vi "Main.vi"() -> ()   [LabVIEW 2020]
doc: "This template is for the Queued Message Handler design pattern.\n\nThe Event Handling Loop generates messages based on user interface actions.\n\nThe Message Handling Loop processes messages generated by the Event Handling Loop, or by other messages. The messages are string values, so new messages can be added easily to the Message Cases case structure in the Message Handling Loop. Each message cluster can also provide an optional value for Message Data, which is a variant that can be converted to whatever message-specific data is required."
uses:
  controls/UI Data.ctl
  support/Message Queue/Message Cluster.ctl
  <vilib>/DAQmx/read.llb/DAQmx Read (Analog 1D DBL 1Chan NSamp).vi
  <extravilib>/ChannelInstances/Messenger-t'Message Queue.lvlib-Message Cluster.ctl'/Write With Abort.vi
  <extravilib>/ChannelInstances/Messenger-t'Message Queue.lvlib-Message Cluster.ctl'/Instantiate.vi
  <extravilib>/ChannelInstances/Messenger-t'Message Queue.lvlib-Message Cluster.ctl'/Endpoint.vi
  <extravilib>/ChannelInstances/Event Messenger-bool/Instantiate.vi
  <extravilib>/ChannelInstances/Event Messenger-bool/))Channel.vi
  <vilib>/DAQmx/create/channels.llb/DAQmx Create Channel (AI-Voltage-Basic).vi
  <vilib>/DAQmx/configure/timing.llb/DAQmx Timing (Sample Clock).vi
  <vilib>/DAQmx/miscellaneous.llb/DAQmx Fill In Error Info.vi
  <vilib>/ErrorRing/Error Ring.xnode
  <extravilib>/ChannelInstances/Event Messenger-bool.lvlib
  support/Message Queue/Message Queue.lvlib
  <extravilib>/ChannelInstances/Messenger-t'Message Queue.lvlib-Message Cluster.ctl'.lvlib
  <resource>/objmgr/daqmx.rc
panel:
  out "Actual Sample Rate":dbl
  in  "Threshold":dbl=4.0
  in  "Analyze Signal":bool
  in  "Sample Rate":dbl=1000.0
  in  "Generate Signal":bool
  out "Threshold Exceeded?":bool
  out "RMS Result":dbl
  out "Current Consumer State":string
  out "Waveform Graph":dbl[](graph)
  in  "Exit":bool
  # "These controls have associated \"Value Changed\" events configured in the Event Structure on the diagram.\n\nReplace them (and reconfigure the Event Structure) with the controls you need for your application."
  # "This template is for the Queued Message Handler design pattern.\n\nSee the block diagram for more information on how to use this template."
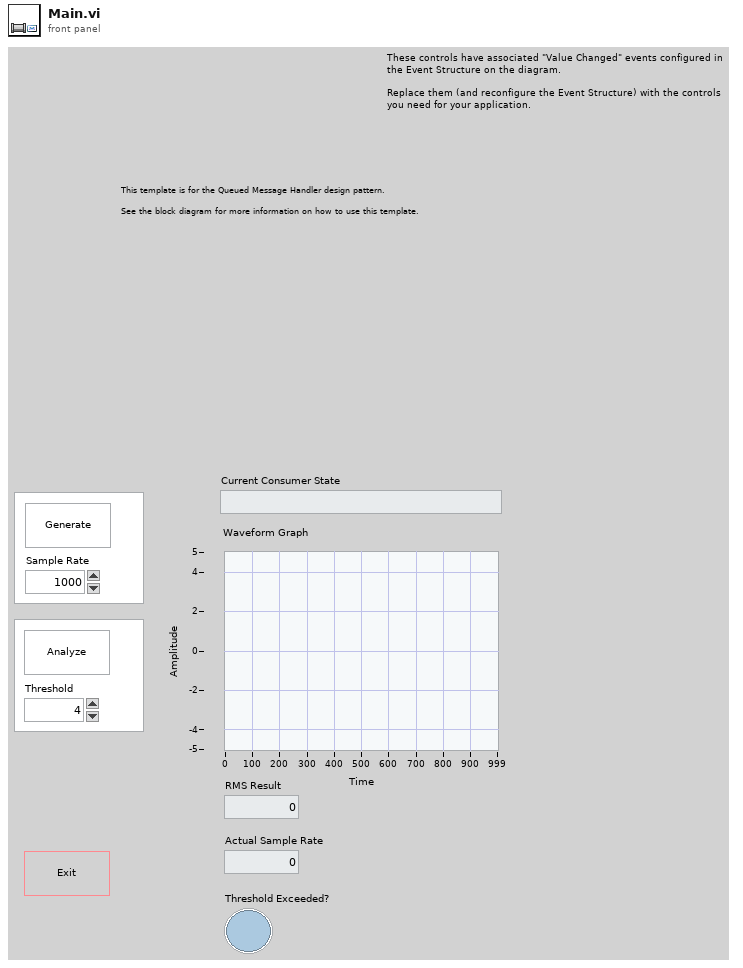
[diagram p1: front panel]
types:
  T1 = typedef "Message Queue.lvlib/Message Cluster.ctl" = cluster{"Message":string, "Message Data":variant}
  T2 = typedef "UI Data.ctl" = cluster{"Message":string, "Message Data":u32}
  T3 = typedef "Messenger-t'Message Queue.lvlib-Message Cluster.ctl'.lvlib/))Channel.ctl" = refnum<queue>
  T4 = typedef "Event Messenger-bool.lvlib/))Channel.ctl" = refnum<queue>
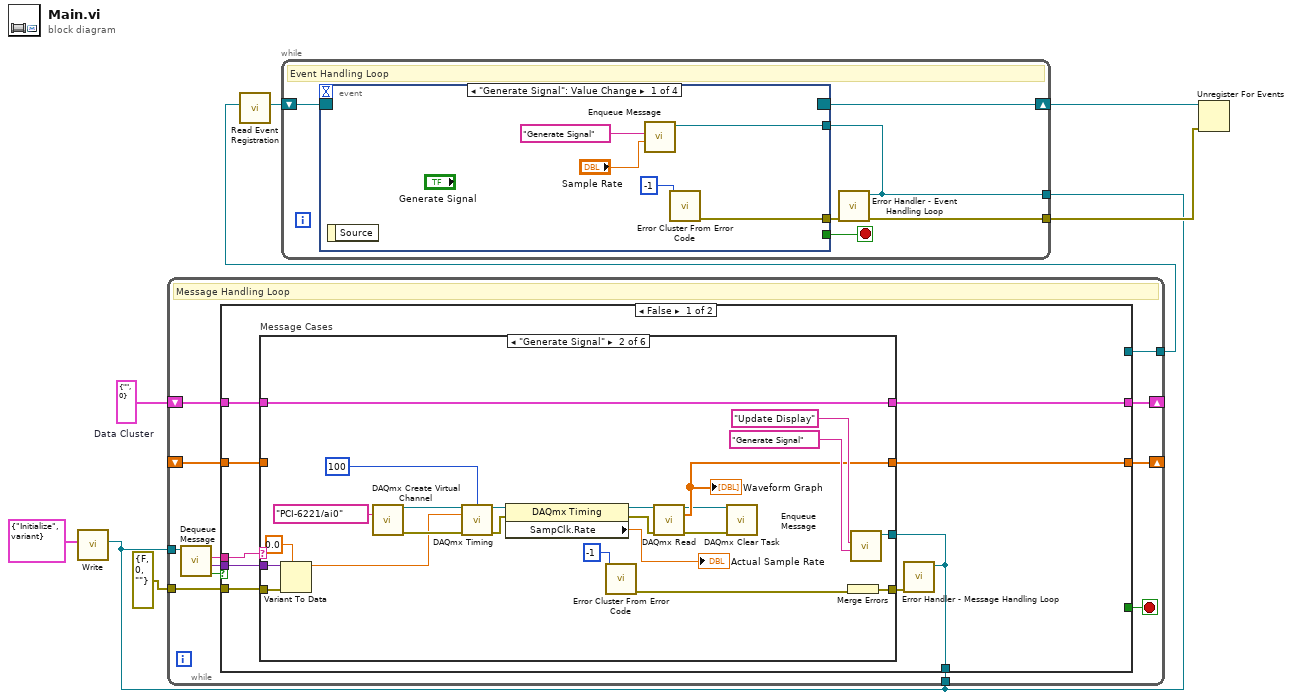
[diagram p0: block diagram]
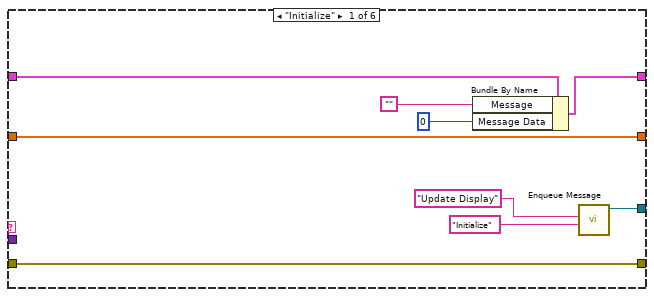
[diagram p2: hidden frame]
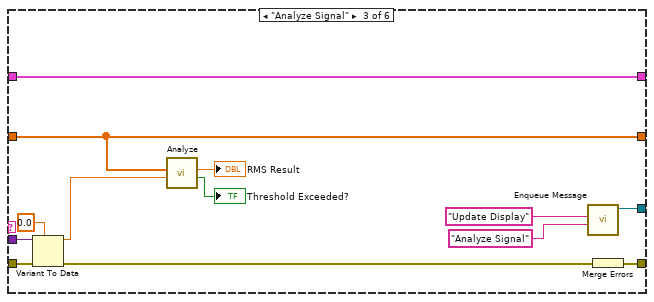
[diagram p3: hidden frame]
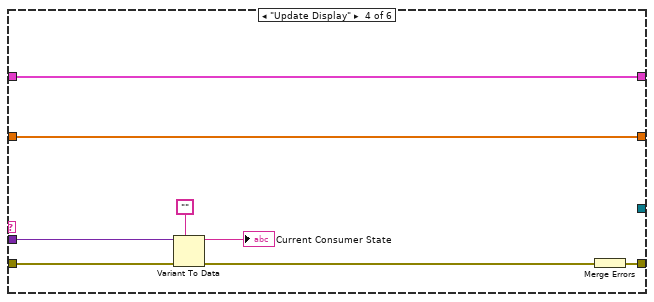
[diagram p4: hidden frame]
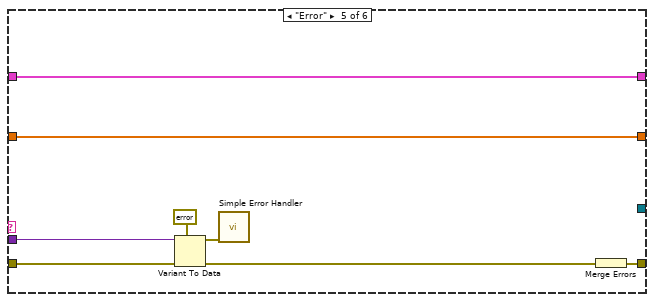
[diagram p5: hidden frame]
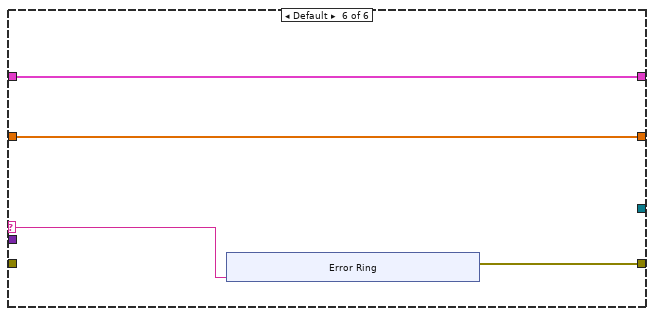
[diagram p6: hidden frame]
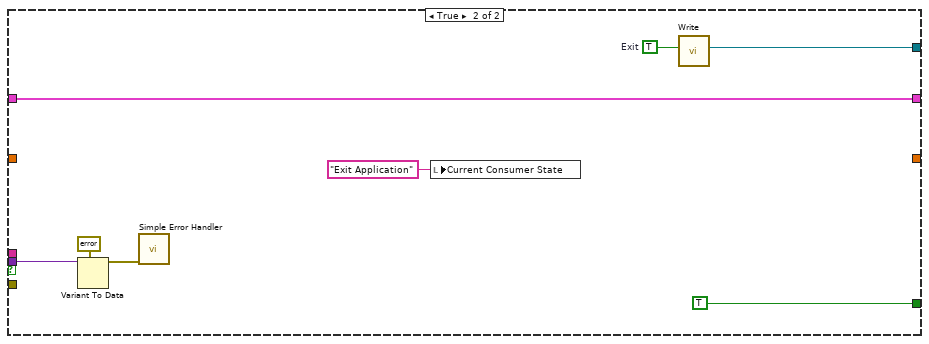
[diagram p7: hidden frame]
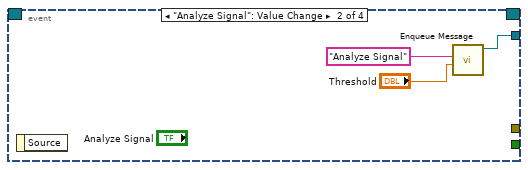
[diagram p8: hidden frame]
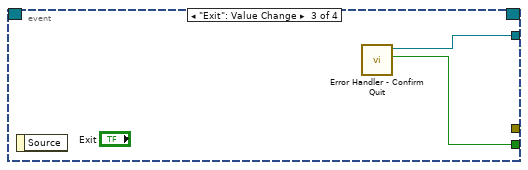
[diagram p9: hidden frame]
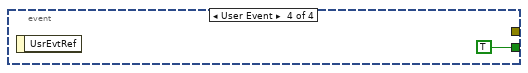
[diagram p10: hidden frame]
diagram:
  w7 = T2 {"Message"="", "Message Data"=0}  # Data Cluster
  n1 = call <extravilib>:"Write.vi"("element"=T1 {"Message"="Initialize", "Message Data"=variant}) -> ("channel"=w2:T3)  [unwired: 8 in, 2 out]
  n2 = while {
    shift-right: [w19] -> _
    shift-left: w7 -> [w20]
    tunnel: [w17] -> w5
    tunnel: w2 -> [w14]
    tunnel: errorcluster {"status"=FALSE, "code"=0, "source"=""} ("error IO") -> [w16]
    tunnel: w2 -> [w15]
    shift-right: [w10] -> _
    shift-left: _ -> [w9]
    stop <- w18 stop-if-true
    # "Message Handling Loop"
    n3 = call "Dequeue Message.vi"("channel"=w14) -> ("channel aborted"=w11:bool, "message data"=w12:variant, "message"=w13:string)  [unwired: 8 in]
    n4 = case shown="False" w11 {
      tunnel: w20 -> [w29 w108]
      tunnel: [w28 w108] -> w19
      tunnel: [_ TRUE] -> w18
      tunnel: [_ w103] -> w17
      tunnel: w13 -> [w26 _]
      tunnel: w12 -> [w25 w105]
      tunnel: w16 -> [w24 _]
      tunnel: [w23 _] -> w15
      tunnel: [w22 _] -> w10
      tunnel: w9 -> [w21 _]
      frame False {
        n5 = case "Message Cases" shown="\"Generate Signal\"" w26 {
          selector: w26 -> [_ _ _ _ _ w92]
          tunnel: w24 -> [w36 w47 w66 w80 w90 _]
          tunnel: [w36 w60 w73 w81 w84 w93] -> w27
          tunnel: w29 -> [w38 w61 w74 w82 w89 w94]
          tunnel: [w37 w61 w74 w82 w89 w94] -> w28
          tunnel: w25 -> [_ w49 w65 w79 w88 _]
          tunnel: [w33 w59 w72 _ _ _] -> w23
          tunnel: [w30 w56 w68 w76 w83 w91] -> w22
          tunnel: w21 -> [w30 _ w68 w76 w83 w91]
          frame "Initialize" {
            # "Initialize - All initialization work should take place in this message, since other loops can potentially enqueue messages that execute immediately after this one."
            n6 = Bundle By Name(cluster=w38, "Message"="", "Message Data"=u32 0 ("Numeric <Replace Me>")) -> (w37:T2)
            n7 = call "Enqueue Message.vi"("data (empty)"="Initialize" ("Initial Message"), "message"="Update Display" ("Message")) -> ("channel"=w33:T3)  [unwired: 9 in]
          }
          frame "Generate Signal" {
            # "Something - Replace this message with functionality for your own application."
            n8 = Variant To Data(error in=w47, type=0.0, Variant=w49) -> (data=w46:dbl)  [unwired: 1 out]
            n9 = call-poly <vilib>:"DAQmx Create Virtual Channel.vi"("physical channels"=tag "PCI-6221/ai0") -> ("task out"=w55:refnum<k21>, "error out"=w54:errorcluster)  [unwired: 13 in]
            n10 = call-poly <vilib>:"DAQmx Timing.vi"("task/channels in"=w55, "samples per channel"=100, "rate"=w46, "error in"=w54) -> ("task out"=w45:refnum<k21>, "error out"=w44:errorcluster)  [unwired: 10 in]
            n11 = property class="DAQmx Timing"(reference=w45, error in=w44) -> (reference out=w43:refnum<k21>, error out=w42:errorcluster, "SampClk.Rate"=→"Actual Sample Rate":dbl)
            n12 = call <vilib>:"Error Cluster From Error Code.vi"("error code (0)"=-1) -> ("error out"=w39:errorcluster)  [unwired: 8 in]
            n13 = call-poly <vilib>:"DAQmx Read.vi"("task/channels in"=w43, "error in"=w42) -> ("task out"=w53:refnum<k21>, "data"=w56:dbl[], "error out"=w52:errorcluster)  [unwired: 11 in]
            "Waveform Graph" <- w56
            n14 = call <vilib>:"DAQmx Clear Task.vi"("task in"=w53, "error in"=w52) -> ()  [unwired: 13 in, 1 out]
            n15 = Merge Errors(w39) -> (w60:errorcluster)
            n16 = call "Enqueue Message.vi"("data (empty)"="Generate Signal" ("\"Do Something\" button pressed"), "message"="Update Display" ("Message")) -> ("channel"=w59:T3)  [unwired: 9 in]
          }
          frame "Analyze Signal" {
            # "Something Else - Replace this message with functionality for your own application."
            n17 = Variant To Data(error in=w66, type=0.0, Variant=w65) -> (data=w63:dbl, error out=w64:errorcluster)
            n18 = call "Analyze.vi"("Threshold (rms)"=w63, "Data (1D DBL)"=w68) -> ("Threshold Exceeded?"=→"Threshold Exceeded?":bool, "RMS Result"=→"RMS Result":dbl)  [unwired: 8 in]
            n19 = call "Enqueue Message.vi"("data (empty)"="Analyze Signal" ("\"Do Something Else\" button pressed"), "message"="Update Display" ("Message")) -> ("channel"=w72:T3)  [unwired: 9 in]
            n20 = Merge Errors(w64) -> (w73:errorcluster)
          }
          frame "Update Display" {
            # "Update Display - Convert the message data to a string to display in the Data Display indicator."
            n21 = Variant To Data(error in=w80, type="", Variant=w79) -> (data=→"Current Consumer State":string, error out=w77:errorcluster)
            n22 = Merge Errors(w77) -> (w81:errorcluster)
          }
          frame "Error" {
            # "Error - Display an error dialog. This message is sent by the \"Error Handler\" VIs at the end of other loops in this application."
            n23 = Variant To Data(error in=w90, type=errorcluster {"status"=FALSE, "code"=0, "source"=""} ("error constant"), Variant=w88) -> (data=w86:errorcluster, error out=w85:errorcluster)
            n24 = call <vilib>:"Simple Error Handler.vi"("error in (no error)"=w86) -> ()  [unwired: 4 in, 5 out]
            n25 = Merge Errors(w85) -> (w84:errorcluster)
          }
          frame Default {
            # "'Default' case only runs if there is a message that isn't defined in any of the other cases.  Output a programming error."
            n26 = xnode "Error Ring"("parameter 0"=w92) -> ("error out"=w93:errorcluster)
          }
        }
        n27 = call "Error Handler - Message Handling Loop.vi"("channel"=w23, "error in (no error)"=w27) -> ()  [unwired: 9 in, 1 out]
      }
      frame True {
        w104 = TRUE  # Exit
        n28 = Variant To Data(type=errorcluster {"status"=FALSE, "code"=0, "source"=""} ("error constant"), Variant=w105) -> (data=w106:errorcluster)  [unwired: 1 in, 1 out]
        n29 = call <vilib>:"Simple Error Handler.vi"("error in (no error)"=w106) -> ()  [unwired: 4 in, 5 out]
        n30 = local write "Current Consumer State"("Exit Application" ("Exit Application")) -> ()
        n31 = call <extravilib>:"Write.vi"("element"=w104) -> ("channel"=w103:T4)  [unwired: 9 in, 1 out]
      }
    }
  }
  n32 = call <extravilib>:"Read Event Registration.vi"("channel"=w5) -> ("event registration refnum"=w4:refnum<event-registration>)  [unwired: 10 in]
  n33 = while {
    shift-right: [w114] -> w8
    shift-left: w4 -> [w115]
    tunnel: [w112] -> w6
    tunnel: w2 -> [w111]
    stop <- w113 stop-if-true
    # "Event Handling Loop"
    n34 = event shown="[0] \"Generate Signal\": Value Change" {
      selector: w115 -> [_ _ _ _]
      dyn-events: [_ _ _ _] -> w114
      timeout: _ -> [_ _ _ _]
      tunnel: [_ _ w124 TRUE ("Discard?")] -> w113
      tunnel: [w120 w123 w125 _] -> w111
      tunnel: [w116 _ _ _] -> w110
      event "Generate Signal": Value Change {
        n35 = event-data() -> ()  [unwired: 1 in, 1 out]
        n36 = call "Enqueue Message.vi"("data (empty)"="Sample Rate", "message"="Generate Signal" ("Message")) -> ("channel"=w120:T3)  [unwired: 9 in]
        n37 = call <vilib>:"Error Cluster From Error Code.vi"("error code (0)"=-1) -> ("error out"=w116:errorcluster)  [unwired: 8 in]
      }
      event "Analyze Signal": Value Change {
        n38 = event-data() -> ()  [unwired: 1 in, 1 out]
        n39 = call "Enqueue Message.vi"("data (empty)"="Threshold", "message"="Analyze Signal" ("Message")) -> ("channel"=w123:T3)  [unwired: 9 in]
      }
      event "Exit": Value Change {
        n40 = event-data() -> ()  [unwired: 1 in, 1 out]
        n41 = call "Error Handler - Confirm Quit.vi"() -> ("exit confirmed"=w124:bool, "channel"=w125:T3)  [unwired: 10 in]
      }
      event User Event {
        n42 = event-data() -> ()  [unwired: 1 in, 1 out]
      }
    }
    n43 = call "Error Handler - Event Handling Loop.vi"("channel"=w111, "error in (no error)"=w110) -> ("dup error in"=w112:errorcluster)  [unwired: 9 in]
  }
  n44 = Unregister For Events(event registration refnum=w8, error in=w6) -> ()  [unwired: 1 out]
